vi "Configure Setpoint.vi"(7 "unit (capacity unit)":u16(ring) items=["capacity unit", "%"], 8 "error in (no error)":errorcluster, 9 "setpoint":sgl, 10 "node address (same)":u8, 11 "ProPar in":refnum<class "PL Bronkhorst ProPar.lvclass">) -> (0 "error out":errorcluster, 3 "ProPar out":refnum<class "PL Bronkhorst ProPar.lvclass">)   [LabVIEW 2015, in "PL Bronkhorst ProPar.lvclass"]
doc: "Configures setpoint of the specified <b>node</b>."
uses:
  PL Bronkhorst ProPar.lvclass
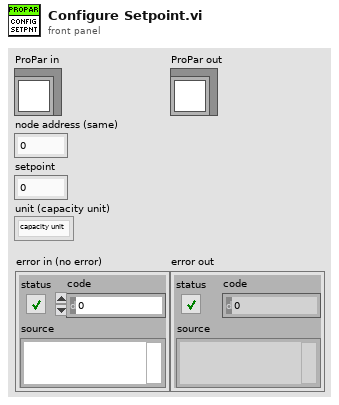
[diagram p1: front panel]
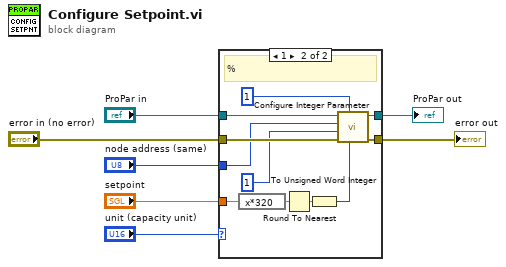
[diagram p0: block diagram]
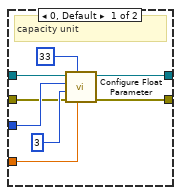
[diagram p2: hidden frame]
diagram:
  n1 = case shown="1" "unit (capacity unit)" {
    tunnel: [w14 w25] -> w7
    tunnel: [w13 w26] -> w6
    tunnel: "ProPar in" -> [w12 w23]
    tunnel: "node address (same)" -> [w11 w22]
    tunnel: "setpoint" -> [w9 w20]
    tunnel: "error in (no error)" -> [w8 w24]
    frame 0, Default {
      # "capacity unit"
      n2 = call "Configure Float Parameter.vi"("value"=w9, "process number"=u8 33, "error in (no error)"=w8, "parameter number"=u8 3 ("process number"), "node"=w11, "ProPar in"=w12) -> ("error out"=w14:errorcluster, "ProPar out"=w13:refnum<class "PL Bronkhorst ProPar.lvclass">)  [unwired: 4 in]
    }
    frame 1 {
      # "%"
      n3 = expression code="x*320"(w20) -> (w18:sgl)
      n4 = Round To Nearest(number=w18) -> (nearest integer value=w17:sgl)
      n5 = To Unsigned Word Integer(number=w17) -> (unsigned 16bit integer=w16:u16)
      n6 = call "Configure Integer Parameter.vi"("value"=w16, "process number"=u8 1, "error in (no error)"=w24, "parameter number"=u8 1 ("process number"), "node"=w22, "ProPar in"=w23) -> ("error out"=w25:errorcluster, "ProPar out"=w26:refnum<class "PL Bronkhorst ProPar.lvclass">)  [unwired: 4 in]
    }
  }
  "ProPar out" <- w6
  "error out" <- w7
